vi "(SubVI)Update Trigger Control Cluster.vi"(8 "error in (no error)":errorcluster caption="에러 입력(에러 없음)", 11 "Trig Ctrl Ref":refnum<vi>) -> (0 "error out":errorcluster caption="에러 출력", 3 "Disable":T1(ring))   [LabVIEW 2020]
uses:
  System Command/Controls/(Ctrl)System Command_Trig GPIO Control.ctl
panel:
  # "Trigger"
  # "L (us)"
  # "H (us)"
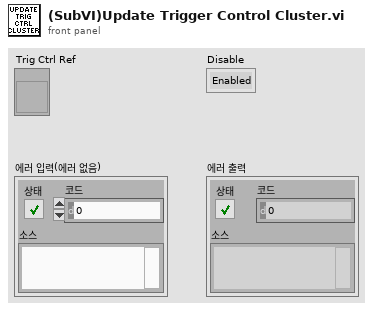
[diagram p1: front panel]
types:
  T1 = enum8{"Enabled", "Disabled", "Disabled and Grayed Out"}
  T2 = typedef "(Ctrl)System Command_Trig GPIO Control.ctl" = cluster{"1st Trig":cluster{"Trigger":bool, "Low":u16, "High":u16}, "2nd Trig":cluster{"Trigger":bool, "Low":u16, "High":u16}, "3rd Trig":cluster{"Trigger":bool, "Low":u16, "High":u16}, "4th Trig":cluster{"Trigger":bool, "Low":u16, "High":u16}}
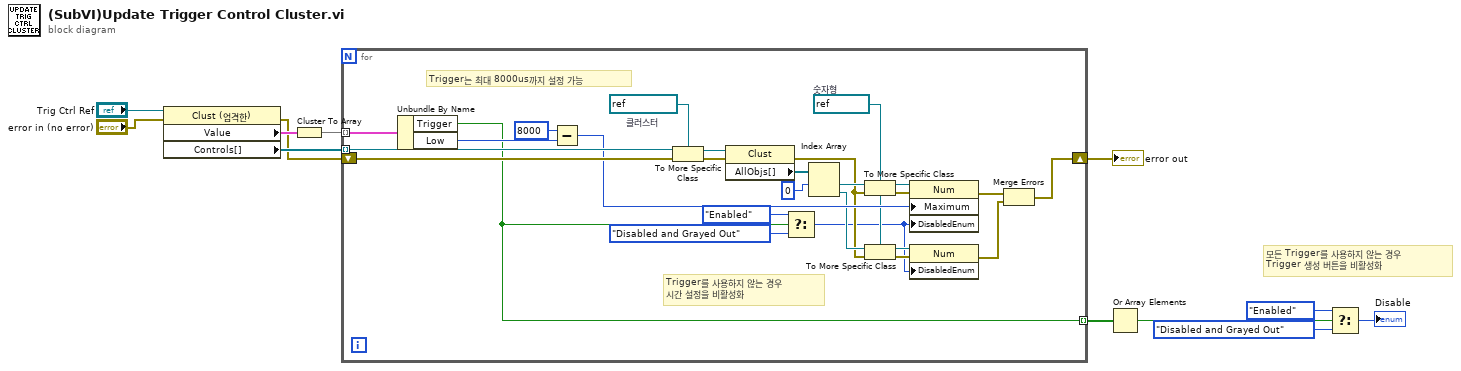
[diagram p0: block diagram]
diagram:
  # "모든 Trigger를 사용하지 않는 경우\nTrigger 생성 버튼을 비활성화"
  n1 = property class="Clust (엄격한)"(reference="Trig Ctrl Ref", error in="error in (no error)") -> (error out=w7:errorcluster, "Value"=w11:T2, "Controls[]"=w9:refnum<vi>[])  [unwired: 1 out]
  n2 = Cluster To Array(cluster=w11) -> (array=w10:cluster{"Trigger":bool, "Low":u16, "High":u16}[])
  n3 = for {
    tunnel: w10 -> [w38] mode=indexing
    tunnel: w9 -> [w35] mode=indexing
    shift-right: [w18] -> w6
    shift-left: w7 -> [w37]
    tunnel: [w14] -> w5 mode=indexing
    w22 = refnum<vi> refnum  # 숫자형
    w33 = refnum<vi> refnum  # 클러스터
    # "Trigger는 최대 8000us까지 설정 가능"
    # "Trigger를 사용하지 않는 경우\n시간 설정을 비활성화"
    n4 = Unbundle By Name(w38) -> ("Trigger"=w14:bool, "Low"=w25:u16)
    n5 = Subtract(x=u16 8000, y=w25) -> (x-y=w28:u16)
    n6 = To More Specific Class(target class=w33, reference=w35, error in=w37) -> (specific class reference=w34:refnum<vi>, error out=w36:errorcluster)
    n7 = property class="Clust"(reference=w34, error in=w36) -> (error out=w21:errorcluster, "AllObjs[]"=w32:refnum<vi>[])  [unwired: 1 out]
    n8 = Select(t=T1."Enabled" ("비활성화"), s=w14, f=T1."Disabled and Grayed Out") -> (s? t:f=w13:T1)
    n9 = Index Array(array=w32, index #1=0 ("인덱스")) -> (element #1=w31:refnum<vi>, element #2=w23:refnum<vi>)  [unwired: 1 in]
    n10 = To More Specific Class(target class=w22, reference=w31, error in=w21) -> (specific class reference=w30:refnum<vi>, error out=w29:errorcluster)
    n11 = To More Specific Class(target class=w22, reference=w23, error in=w21) -> (specific class reference=w19:refnum<vi>, error out=w20:errorcluster)
    n12 = property class="Num"(reference=w30, error in=w29, "Maximum"=w28, "DisabledEnum"=w13) -> (error out=w27:errorcluster)  [unwired: 1 out]
    n13 = property class="Num"(reference=w19, error in=w20, "DisabledEnum"=w13) -> (error out=w17:errorcluster)  [unwired: 1 out]
    n14 = Merge Errors(w27, w17) -> (w18:errorcluster)
  }
  "error out" <- w6
  n15 = Or Array Elements(Boolean array=w5) -> (logical OR=w4:bool)
  n16 = Select(t=T1."Enabled" ("비활성화"), s=w4, f=T1."Disabled and Grayed Out") -> (s? t:f=→"Disable":T1)
